vi "17_09_20199_49am.vi"() -> ()   [LabVIEW 2017]
uses:
  <vilib>/Simulation/Scripting/Companion Diagram/SimConfigNode/SimParams.ctl
  <vilib>/Simulation/Scripting/Companion Diagram/SimConfigNode/_simSolvers.ctl
  <vilib>/Simulation/Implementation/Shared/SIMSCR Execution Mode.ctl
  <vilib>/Simulation/Param Hierarchy/Typedefs/SIMPH Param Control Actions.ctl
  <vilib>/Simulation/Implementation/Shared/NILVSim_ParamChanged.vi
  <vilib>/Simulation/Implementation/Shared/NILVSIM_BeginStep.vi
  <vilib>/Simulation/Implementation/Shared/NILVSim_Manager.vi
  <vilib>/Utility/error.llb/Clear Errors.vi
  <vilib>/Simulation/Implementation/Shared/NILVSim_FinalizeModel.vi
  <vilib>/DAQmx/read.llb/DAQmx Read (Counter DBL 1Chan 1Samp).vi
  <vilib>/DAQmx/read.llb/DAQmx Read (Digital Bool 1Line 1Point).vi
  917b7e52-755f-4d44-bea8-9e7c9beac24e.vi
  a58f9967-76f1-4ebc-ad3d-26e75a3ca160.vi
  <vilib>/DAQmx/write.llb/DAQmx Write (Analog DBL 1Chan 1Samp).vi
  <vilib>/DAQmx/create/channels.llb/DAQmx Create Channel (AO-Voltage-Basic).vi
  <vilib>/DAQmx/create/channels.llb/DAQmx Create Channel (DI-Digital Input).vi
  <vilib>/DAQmx/create/channels.llb/DAQmx Create Channel (CI-Count Edges).vi
  <vilib>/Simulation/Implementation/Shared/SIM Unbundle Sim Info.vi
  <vilib>/Simulation/Implementation/Shared/NILVSim_Initialize.vi
  <vilib>/Simulation/Utility/Implementation/NILVSim Get Time and IsAcceptedStep.vi
  <vilib>/Simulation/Implementation/Shared/SIMSH Read Queue.vi
  <vilib>/Simulation/Implementation/Shared/NILVSim_GetModelError.vi
  <vilib>/Simulation/Implementation/Shared/SIM Bundle Sim Info.vi
  Global pulses.vi
  <vilib>/DAQmx/miscellaneous.llb/DAQmx Fill In Error Info.vi
  <vilib>/Simulation/Implementation/XNodeFramework/SimXNode/SimX.xnode
  <vilib>/Simulation/Model Libraries/PID/SIM PID (Parallel).vi
  <vilib>/Simulation/Model Libraries/PID/SIM PID.vi
  <vilib>/Simulation/Scripting/Companion Diagram/SimConfigNode/SimDog.xnode
  <vilib>/Simulation/Model Libraries/PID/SIM PID (Academic).vi
  <vilib>/Simulation/Implementation/Shared/NI_SIM_Implementation.lvlib
panel:
  out "Numeric 2":dbl
  out "swiches pressed y":dbl
  out "swiches pressed x":dbl
  in  "Reset":bool
  out "time":dbl
  out "frequency (moving)":dbl
  out "switch dir":dbl
  out "swiches":bool
  out "Boolean 2":bool
  in  "rectangle":bool
  in  "stage rectangle":T1(ring)
  out "stay1":dbl
  out "stay":dbl
  out "calculating error x":dbl
  out "calculating error y":dbl
  in  "origin":bool
  out "Previous Y":dbl
  out "Previous X":dbl
  out "Current Y":dbl
  out "Current X":dbl
  out "previous index":dbl
  out "both/reset enter":bool
  out "reset complete":bool
  out "x circle":bool
  out "y circle":bool
  out "Point circle is drawing":dbl
  out "false":bool
  in  "Radius 2":dbl
  out "No of Points":dbl
  out "Passing Y":dbl
  out "Y array":dbl[](array[numeric])
  out "array Y length 2":dbl
  out "Passing X":dbl
  out "X array":dbl[](array[numeric])
  out "array x Length 2":dbl
  in  "stage circle":T2(ring)
  in  "check instruc":bool
  out "x entered":dbl
  out "y enetred":dbl
  out "greater -1 x":bool
  out "less 1 x":bool
  out "direction selected":dbl
  out "Shape drawing steps":enum16{"corner", "1st switch", "reverse"}(ring)
  in  "height":dbl
  in  "length":dbl
  in  "Has encoders been reset?":enum16{"don't reset", "reset"}(ring)
  out "x distance currently being travelled":dbl
  out "y distance currently being travelled":dbl
  out "error calced":dbl
  out "p1 dis 2":dbl
  out "p1 dis":dbl
  out "error y":dbl
  out "calc distance y":dbl
  out "calc distanc x":dbl
  out "error x":dbl
  out "reached y":bool
  out "reached x":bool
  out "Numeric":dbl
  out "In drawing mode":bool
  in  "Right-Down":bool
  in  "Left-Up":bool
  in  "Left-Down":bool
  in  "Right-Up":bool
  in  "right":bool
  in  "left":bool
  in  "motor 2":dbl(slide)=1.5 scale=-10.0..10.0
  in  "down":bool
  in  "up":bool
  in  "Y Length":dbl=30.0
  in  "X Length":dbl=30.0
  in  "Motor 2 encoder":tag="Dev1/ctr1"
  out "Pulses M2":dbl format="%.2f"
  in  "Motor 1 encoder":tag="Dev1/ctr0"
  out "Pulses M1":dbl format="%.2f"
  out "Right":bool
  out "Bottom":bool
  out "Left":bool
  out "Top":bool
  in  "Switch 4/Line 3":tag="Dev1/port0/line3"
  in  "Switch 3/Line 2":tag="Dev1/port0/line2"
  in  "Switch 2/Line 1":tag="Dev1/port0/line1"
  in  "Switch 1/Line 0":tag="Dev1/port0/line0"
  in  "Motor stop":bool
  in  "Motor 1":tag="Dev1/ao0"
  in  "max Voltage":dbl=10.0
  in  "Min Voltage":dbl=-10.0
  in  "Motor 2":tag="Dev1/ao1"
  in  "motor 1":dbl(slide)=1.5 scale=-10.0..10.0
  in  "stop":bool
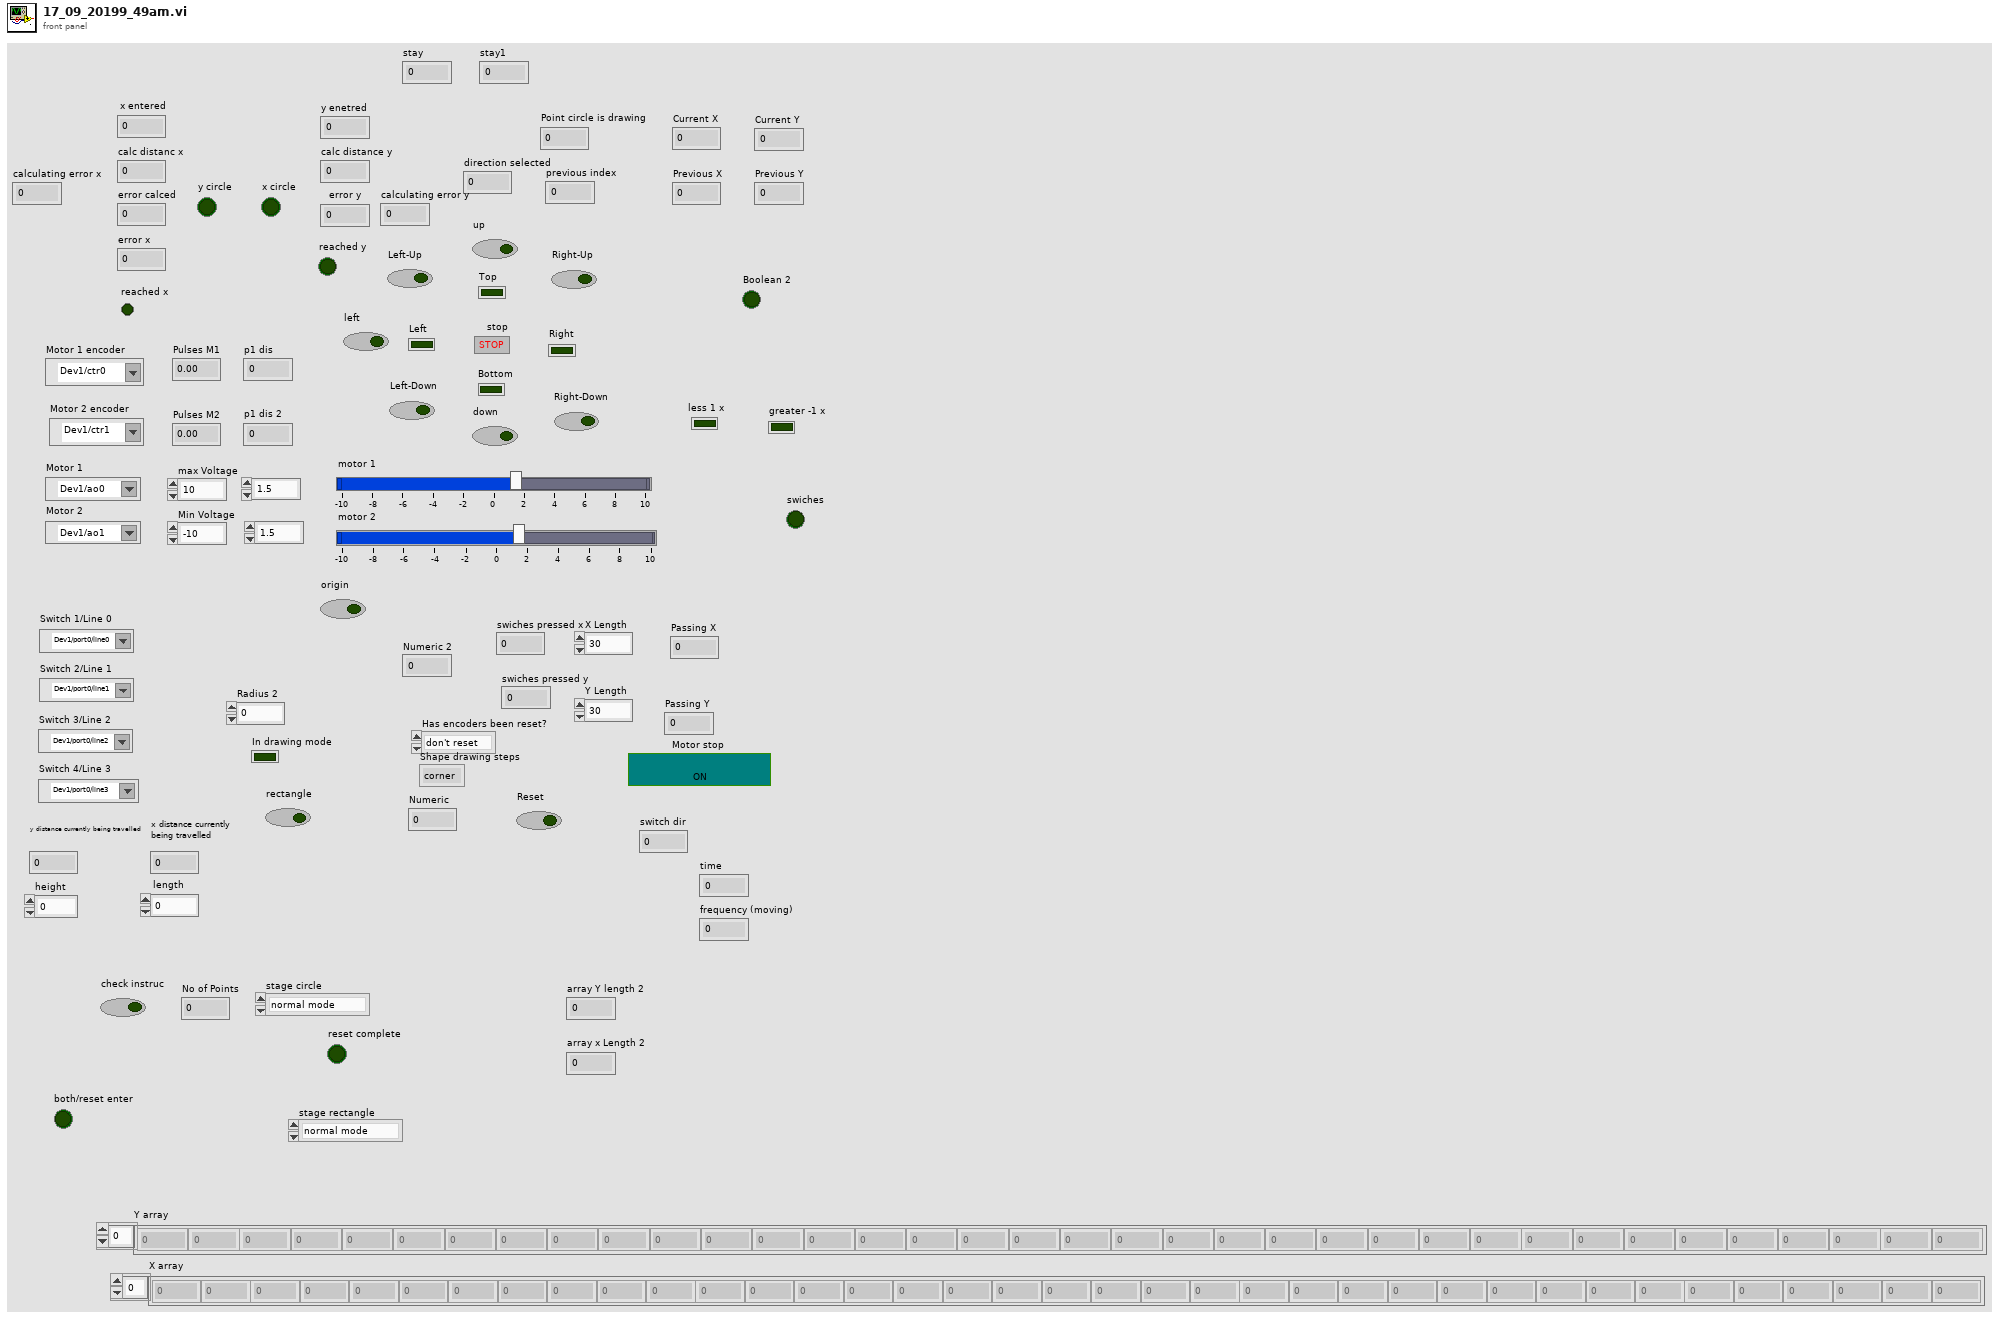
[diagram p1: front panel]
types:
  T1 = enum16{"normal mode", "take to origin", "reset before start", "reset before right", "giving values right", "drawing right", "reset before down", "giving values down", "drawing down", "reset before left", "giving value left", "drawing left", "reset before up", "giving values up", "drawing up", "last step"}
  T2 = enum16{"normal mode", "take to origin", "reset before start", "create points", "draw points", "checking if draw", "reset draw counter"}
  T3 = enum16{"Simulate to Completion", "Single Time-Step Simulation (Fixed Step Only)"}
  T4 = typedef "SIMSCR Execution Mode.ctl" = enum16{"Simulate to Completion", "Single Time-Step Simulation (Fixed Step Only)"}
  T5 = typedef "SIMPH Param Control Actions.ctl" = enum16{"get params", "set params"}
  T6 = cluster{"SIMSH Sim Time":dbl, "SIM PID Derivative Gain.vi":cluster{"output":dbl}, "SIM PID Derivative Gain.vi - SIMSH":cluster{"SIMSH Sim Time":dbl, "t 3":dbl, "Select 2":cluster{"s? t:f":dbl}, "Equal?":cluster{"x = y?":bool}, "Or":cluster{"x .or. y?":bool}, "Equal To 0?":cluster{"x = 0?":bool}}, "High Frequency [s] (Tf)":dbl, "Gain":cluster{"output":dbl}, "Summation":cluster{"Result":dbl}, "Integral Gain - series.vi":cluster{"output":dbl}, "Integral Gain - series.vi - SIMSH":cluster{"SIMSH Sim Time":dbl, "Select 2":cluster{"s? t:f":dbl}, "integral in gain?":bool, "Integrator":cluster{"output y(t)":dbl}, "Gain 2":cluster{"output":dbl}, "Select":cluster{"s? t:f":dbl}, "Equal To 0?":cluster{"x = 0?":bool}, "Reciprocal":cluster{"1/x":dbl}}}
  T7 = typedef "SimParams.ctl" = cluster{"Initial Time (s)":dbl, "Final Time (s)":dbl, "Step Size (s)":dbl, "ODE Solver":T8, "Minimum Step Size (s)":dbl, "Maximum Step Size (s)":dbl, "Relative Tolerance":dbl, "Absolute Tolerance":dbl, "Software Timing":bool, "Initial Step Size (s)":dbl, "Automatic Fixed Step Size?":bool, "Automatic Discrete Step Size?":bool, "Discrete Step Size (s)":dbl, "Calculate using Time Step":bool, "Solver Wired?":bool, "Prev.Frm.Expected End":u64, "Prev.Frm.Actual End":u64, "Prev.Frm.Finished Late?":bool, "Prev.Iter.Expected End":u64, "Prev.Iter.Actual End":u64, "Prev.Iter.Finished Late?":bool, "Expected Iteration Start":u64, "Actual Iteration Start":u64, "Expected Frame Start":u64, "Actual Frame Start":u64, "Source Name":string, "Name":string, "Period":i64, "Deadline":i64, "Offset":i64, "Start":i64, "Priority":i32, "Timeout":i32, "Processor":i32, "Mode":enum32{"No Change", "Process missed periods, maintain original phase", "Discard missed periods, maintain original phase", "Process missed periods, ignore original phase", "Discard missed periods, ignore original phase"}, "Wakeup reason":enum32{"Normal", "Aborted", "Asynchronous wakeup", "Timing source error", "Timed loop error", "Timeout"}, "Error":errorcluster, "Source Type":string, "Secondary Source Type":string, "Global End Time":u64, "Global Start Time":u64, "Full Solver Reset":bool, "Execution Mode":T4, "Nan/Inf Check":bool, "Custom Solver Library":string, "Solver Is Variable":bool, "custom solver name":string, "Signal Collection Decimation":u32}
  T8 = typedef "_simSolvers.ctl" = enum16{"Runge-Kutta 1 (Euler)", "Runge-Kutta 2", "Runge-Kutta 3", "Runge-Kutta 4", "Runge-Kutta 23 (variable)", "Runge-Kutta 45 (variable)", "BDF (variable)", "Adams-Moulton (variable)", "Rosenbrock (variable)", "Discrete States Only", "SDIRK 4 (variable)", "Radau 5 (variable)", "Radau 9 (variable)", "Radau 13 (variable)", "Radau [Variable Order] (variable)", "Gear's Method (variable)", "Linearizer", "State Query", "Trim Eval", "Custom Solver"}
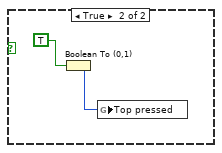
[diagram p2: hidden frame]
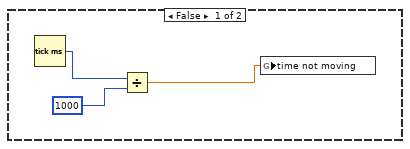
[diagram p6: hidden frame]
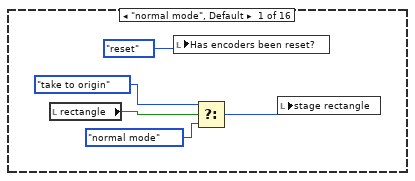
[diagram p8: hidden frame]
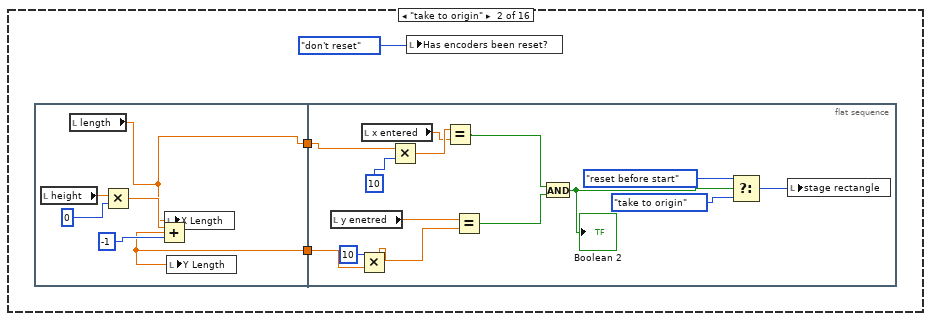
[diagram p9: hidden frame]
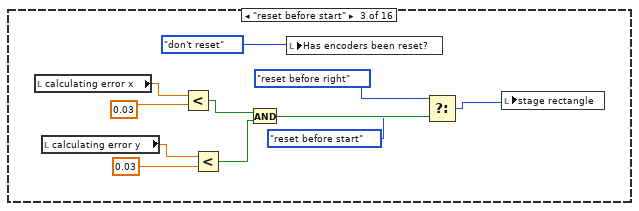
[diagram p10: hidden frame]
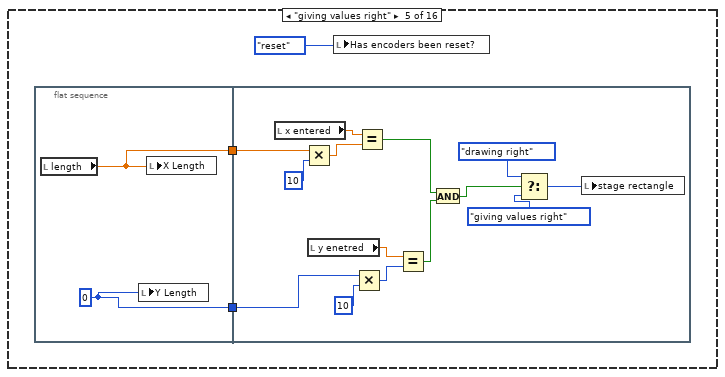
[diagram p11: hidden frame]
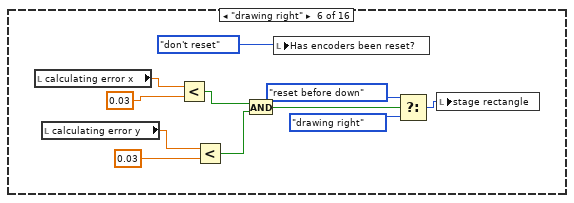
[diagram p12: hidden frame]
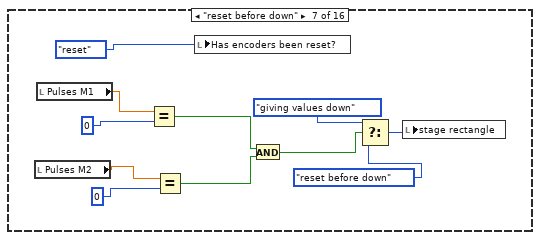
[diagram p13: hidden frame]
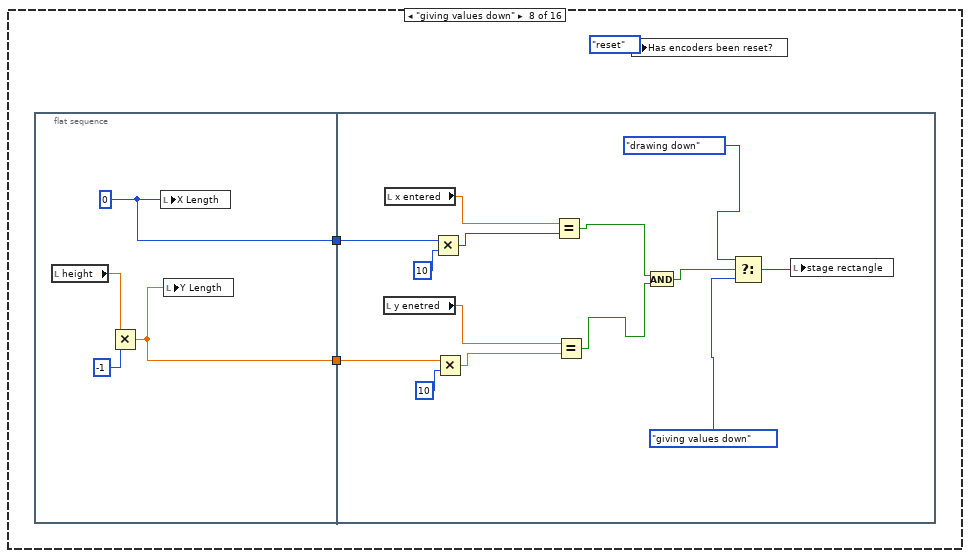
[diagram p14: hidden frame]
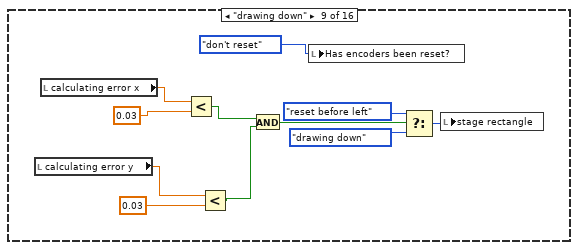
[diagram p15: hidden frame]
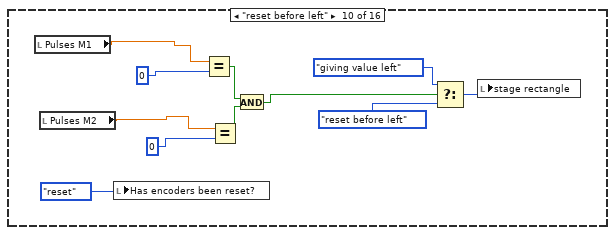
[diagram p16: hidden frame]
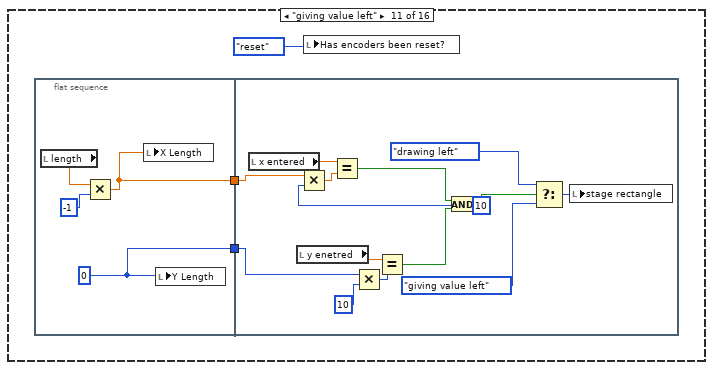
[diagram p17: hidden frame]
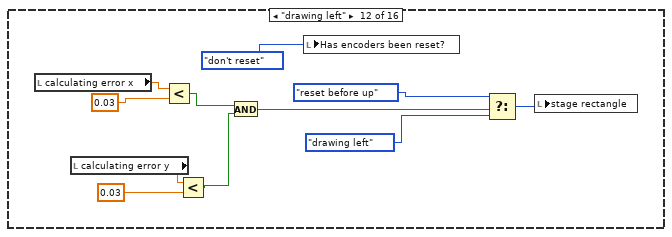
[diagram p18: hidden frame]
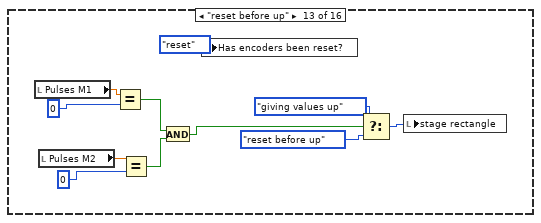
[diagram p19: hidden frame]
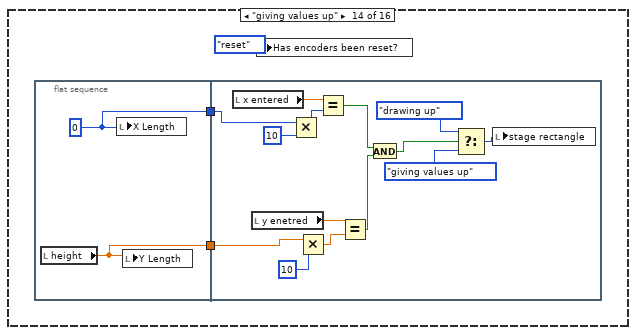
[diagram p20: hidden frame]
diagram:
  n1 = call-poly <vilib>:"DAQmx Create Virtual Channel.vi"("lines"="Switch 1/Line 0") -> ("task out"=w36:refnum<k21>, "error out"=w32:errorcluster)  [unwired: 13 in]
  n2 = call-poly <vilib>:"DAQmx Create Virtual Channel.vi"("lines"="Switch 2/Line 1") -> ("task out"=w35:refnum<k21>, "error out"=w31:errorcluster)  [unwired: 13 in]
  n3 = call-poly <vilib>:"DAQmx Create Virtual Channel.vi"("lines"="Switch 3/Line 2") -> ("task out"=w34:refnum<k21>, "error out"=w30:errorcluster)  [unwired: 13 in]
  n4 = call-poly <vilib>:"DAQmx Create Virtual Channel.vi"("lines"="Switch 4/Line 3") -> ("task out"=w33:refnum<k21>, "error out"=w29:errorcluster)  [unwired: 13 in]
  n5 = call-poly <vilib>:"DAQmx Create Virtual Channel.vi"("maximum value"="max Voltage", "minimum value"="Min Voltage", "physical channels"="Motor 1") -> ("task out"=w46:refnum<k21>, "error out"=w42:errorcluster)  [unwired: 11 in]
  n6 = call <vilib>:"DAQmx Start Task.vi"("task/channels in"=w36, "error in"=w32) -> ("task out"=w28:refnum<k21>, "error out"=w26:errorcluster)  [unwired: 12 in]
  n7 = call <vilib>:"DAQmx Start Task.vi"("task/channels in"=w35, "error in"=w31) -> ("task out"=w24:refnum<k21>, "error out"=w21:errorcluster)  [unwired: 12 in]
  n8 = call-poly <vilib>:"DAQmx Create Virtual Channel.vi"("maximum value"="max Voltage", "minimum value"="Min Voltage", "physical channels"="Motor 2") -> ("task out"=w49:refnum<k21>, "error out"=w41:errorcluster)  [unwired: 11 in]
  n9 = call-poly <vilib>:"DAQmx Create Virtual Channel.vi"("counter"="Motor 1 encoder") -> ("task out"=w7:refnum<k21>, "error out"=w2:errorcluster)  [unwired: 13 in]
  n10 = call-poly <vilib>:"DAQmx Create Virtual Channel.vi"("counter"="Motor 2 encoder") -> ("task out"=w6:refnum<k21>)  [unwired: 13 in, 1 out]
  n11 = call <vilib>:"DAQmx Start Task.vi"("task/channels in"=w34, "error in"=w30) -> ("task out"=w23:refnum<k21>, "error out"=w20:errorcluster)  [unwired: 12 in]
  n12 = call <vilib>:"DAQmx Start Task.vi"("task/channels in"=w33, "error in"=w29) -> ("task out"=w22:refnum<k21>, "error out"=w19:errorcluster)  [unwired: 12 in]
  n13 = call <vilib>:"DAQmx Start Task.vi"("task/channels in"=w7) -> ("task out"=w3:refnum<k21>)  [unwired: 13 in, 1 out]
  n14 = call <vilib>:"DAQmx Start Task.vi"("task/channels in"=w6) -> ("task out"=w1:refnum<k21>)  [unwired: 13 in, 1 out]
  n15 = while {
    tunnel: w49 -> [w249]
    tunnel: [w246] -> w48
    tunnel: w46 -> [w243]
    tunnel: [w242] -> w45
    tunnel: w42 -> [w240]
    tunnel: w41 -> [w239]
    tunnel: w28 -> [w233]
    tunnel: [w232] -> w27
    tunnel: w26 -> [w231]
    tunnel: [w230] -> w25
    tunnel: w24 -> [w229]
    tunnel: w23 -> [w228]
    tunnel: w22 -> [w227]
    tunnel: w21 -> [w226]
    tunnel: w20 -> [w225]
    tunnel: w19 -> [w224]
    tunnel: [w223] -> w18
    tunnel: [w222] -> w17
    tunnel: [w221] -> w16
    tunnel: [w220] -> w15
    tunnel: [w219] -> w14
    tunnel: [w218] -> w13
    tunnel: [w161] -> w10
    tunnel: w3 -> [w163]
    tunnel: w2 -> [w162]
    tunnel: w1 -> [w159]
    stop <- "stop" stop-if-true
    n16 = case shown="True" "check instruc" {
      frame False {
        "false" <- TRUE
      }
      frame True {
        n17 = case shown="\"create points\"" "stage circle" {
          frame "normal mode", Default {
            n18 = local read "check instruc"() -> (w501:bool)
            n19 = local write "Y Length"(0) -> ()
            n20 = local write "X Length"(0) -> ()
            n21 = local write "Has encoders been reset?"(enum16{"don't reset", "reset"}."reset") -> ()
            n22 = Select(t=T2."take to origin", s=w501, f=T2."normal mode") -> (s? t:f=w502:T2)
            n23 = local write "stage circle"(w502) -> ()
          }
          frame "take to origin" {
            n24 = flat-sequence {
              tunnel: [w513] -> w506
              tunnel: [w508] -> w505
              tunnel: w506 -> [w518]
              tunnel: w505 -> [w517]
              frame #0 {
                n25 = local read "Radius 2"() -> (w512:dbl)
                n26 = local read "Radius 2"() -> (w515:dbl)
                n27 = Multiply(x=w512, y=0) -> (x*y=w509:dbl)
                n28 = Multiply(x=w515, y=0) -> (x*y=w513:dbl)
                n29 = Add(x=w509, y=-1) -> (x+y=w508:dbl)
                n30 = local write "Y Length"(w508) -> ()
                n31 = local write "X Length"(w513) -> ()
              }
              frame #1 {
                n32 = Multiply(x=10, y=w517) -> (x*y=w528:dbl)
                n33 = local read "y enetred"() -> (w522:dbl)
                n34 = local read "x entered"() -> (w521:dbl)
                n35 = Multiply(x=10, y=w518) -> (x*y=w527:dbl)
                n36 = Equal?(x=w521, y=w527) -> (x = y?=w524:bool)
                n37 = Equal?(x=w528, y=w522) -> (x = y?=w523:bool)
                n38 = And(x=w524, y=w523) -> (x .and. y?=w529:bool)
                n39 = Select(t=T2."reset before start", s=w529, f=T2."take to origin") -> (s? t:f=w516:T2)
                n40 = local write "stage circle"(w516) -> ()
              }
            }
            n41 = local write "Has encoders been reset?"(enum16{"don't reset", "reset"}."reset") -> ()
          }
          frame "reset before start" {
            n42 = local read "calculating error x"() -> (w539:dbl)
            n43 = local read "calculating error y"() -> (w537:dbl)
            n44 = Less?(x=w539, y=0.01) -> (x < y?=w535:bool)
            n45 = Less?(x=w537, y=0.01) -> (x < y?=w534:bool)
            n46 = local write "Has encoders been reset?"(enum16{"don't reset", "reset"}."don't reset") -> ()
            n47 = And(x=w535, y=w534) -> (x .and. y?=w533:bool)
            n48 = Select(t=T2."create points", s=w533, f=T2."reset before start") -> (s? t:f=w530:T2)
            n49 = local write "stage circle"(w530) -> ()
          }
          frame "create points" {
            n50 = flat-sequence {
              frame #0 {
                n51 = for {
                  N: 36 -> [_]
                  shift-right: [w551] -> w548
                  shift-left: _ -> [_]
                  tunnel: [w551] -> w543 mode=indexing
                  shift-right: [w550] -> w546
                  shift-left: _ -> [_]
                  tunnel: [w550] -> w544 mode=indexing
                  i -> [w552]
                  n52 = Multiply(x=2, y=3.141592653589793) -> (x*y=w555:dbl)
                  n53 = Increment(x=w552) -> (x+1=w553:i32)
                  n54 = Divide(x=w555, y=36) -> (x/y=w557:dbl)
                  n55 = Multiply(x=w557, y=w553) -> (x*y=w554:dbl)
                  n56 = Cosine(x=w554) -> (cos(x)=w560:dbl)
                  n57 = Sine(x=w554) -> (sin(x)=w561:dbl)
                  n58 = Multiply(x=w561, y="Radius 2") -> (x*y=w551:dbl)
                  n59 = Multiply(x=w560, y="Radius 2") -> (x*y=w550:dbl)
                  "No of Points" <- w552
                }
                "Passing Y" <- w548
                "Y array" <- w543
                "Passing X" <- w546
                "X array" <- w544
                n60 = Array Size(array=w543) -> (size(s)=→"array Y length 2":i32)
                n61 = Array Size(array=w544) -> (size(s)=→"array x Length 2":i32)
              }
              frame #1 {
                n62 = local read "Y array"() -> (w568:dbl[])
                n63 = Index Array(array=w568, index=1) -> (element=w569:dbl)
                n64 = local read "X array"() -> (w570:dbl[])
                n65 = Index Array(array=w570, index=1) -> (element=w571:dbl)
                n66 = Insert Into Array(array=w568, index=36, new element=w569) -> (w566:dbl[])
                n67 = Insert Into Array(array=w570, index=36, new element=w571) -> (w567:dbl[])
                n68 = local write "Y array"(w566) -> ()
                n69 = local write "X array"(w567) -> ()
              }
              frame #2 {
                n70 = local read "No of Points"() -> (w576:dbl)
                n71 = Equal?(x=w576, y=35) -> (x = y?=w577:bool)
                n72 = Select(t=T2."draw points", s=w577, f=T2."create points") -> (s? t:f=w575:T2)
                n73 = local write "stage circle"(w575) -> ()
              }
            }
            n74 = local write "Has encoders been reset?"(enum16{"don't reset", "reset"}."don't reset") -> ()
          }
          frame "draw points" {
            n75 = flat-sequence {
              frame #0 {
                n76 = local read "Point circle is drawing"() -> (w606:dbl)
                n77 = local read "previous index"() -> (w598:dbl)
                n78 = local read "Y array"() -> (w599:dbl[])
                n79 = local read "X array"() -> (w600:dbl[])
                n80 = Index Array(array=w599, index=w598) -> (element=→"Previous Y":dbl)
                n81 = Index Array(array=w600, index=w598) -> (element=→"Previous X":dbl)
                n82 = local read "X array"() -> (w601:dbl[])
                n83 = local read "Previous X"() -> (w588:dbl)
                n84 = local read "Current X"() -> (w593:dbl)
                n85 = local read "Y array"() -> (w602:dbl[])
                n86 = local read "Current X"() -> (w591:dbl)
                n87 = Greater Or Equal?(x=w606, y=36) -> (x >= y?=w604:bool)
                n88 = Not Equal To 0?(x=w606) -> (x != 0?=w594:bool)
                n89 = local read "Previous Y"() -> (w589:dbl)
                n90 = local read "Current Y"() -> (w590:dbl)
                n91 = Index Array(array=w601, index=w606) -> (element=→"Current X":dbl)
                n92 = Subtract(x=w591, y=w588) -> (x-y=w586:dbl)
                n93 = Select(t=w586, s=w594, f=w593) -> (s? t:f=w583:dbl)
                n94 = Select(t=T2."normal mode", s=w604, f=T2."draw points") -> (s? t:f=w603:T2)
                n95 = Index Array(array=w602, index=w606) -> (element=→"Current Y":dbl)
                n96 = Subtract(x=w590, y=w589) -> (x-y=w585:dbl)
                n97 = local read "Current Y"() -> (w592:dbl)
                n98 = local write "X Length"(w583) -> ()
                n99 = Not(x=w604) -> (.not. x?=w605:bool)
                n100 = local write "stage circle"(w603) -> ()
                n101 = Not Equal To 0?(x=w606) -> (x != 0?=w595:bool)
                n102 = Select(t=w585, s=w595, f=w592) -> (s? t:f=w584:dbl)
                n103 = local write "Y Length"(w584) -> ()
                n104 = local write "check instruc"(w605) -> ()
              }
              frame #1 {
                n105 = local write "stage circle"(T2."checking if draw") -> ()
              }
            }
            n106 = local write "Has encoders been reset?"(enum16{"don't reset", "reset"}."don't reset") -> ()
          }
          frame "checking if draw" {
            n107 = local read "calculating error x"() -> (w611:dbl)
            n108 = local read "calculating error y"() -> (w609:dbl)
            n109 = local read "Point circle is drawing"() -> (w614:dbl)
            n110 = Greater Or Equal?(x=0.01, y=w611) -> (x >= y?=w617:bool)
            "x circle" <- w617
            n111 = Greater Or Equal?(x=0.01, y=w609) -> (x >= y?=w618:bool)
            "y circle" <- w618
            n112 = And(x=w618, y=w617) -> (x .and. y?=w615:bool)
            "both/reset enter" <- w615
            n113 = Increment(x=w614) -> (x+1=w620:dbl)
            n114 = Select(t=w620, s=w615, f=w614) -> (s? t:f=→"Point circle is drawing":dbl)
            n115 = Select(t=T2."reset draw counter", s=w615, f=T2."checking if draw") -> (s? t:f=w616:T2)
            n116 = local write "stage circle"(w616) -> ()
          }
          frame "reset draw counter" {
            n117 = for {
              N: 1 -> [_]
              i -> [w625]
              n118 = local read "Point circle is drawing"() -> (w630:dbl)
              n119 = local read "Pulses M2"() -> (w635:dbl)
              n120 = local read "Pulses M1"() -> (w636:dbl)
              n121 = Equal To 0?(x=w635) -> (x = 0?=w634:bool)
              n122 = Equal To 0?(x=w636) -> (x = 0?=w632:bool)
              n123 = local read "previous index"() -> (w627:dbl)
              n124 = local write "Has encoders been reset?"(enum16{"don't reset", "reset"}."reset") -> ()
              n125 = And(x=w632, y=w634) -> (x .and. y?=w633:bool)
              n126 = Subtract(x=w630, y=1) -> (x-y=w628:dbl)
              n127 = Select(t=T2."draw points", s=w633, f=T2."reset draw counter") -> (s? t:f=w637:T2)
              n128 = Equal To 0?(x=w625) -> (x = 0?=w624:bool)
              n129 = local write "stage circle"(w637) -> ()
              n130 = Select(t=w628, s=w624, f=w627) -> (s? t:f=→"previous index":dbl)
              "reset complete" <- TRUE
            }
          }
        }
      }
    }
    n131 = case shown="True" "rectangle" {
      frame False {
      }
      frame True {
        n132 = case shown="\"reset before right\"" "stage rectangle" {
          frame "normal mode", Default {
            n133 = local read "rectangle"() -> (w290:bool)
            n134 = local write "Has encoders been reset?"(enum16{"don't reset", "reset"}."reset") -> ()
            n135 = Select(t=T1."take to origin", s=w290, f=T1."normal mode") -> (s? t:f=w288:T1)
            n136 = local write "stage rectangle"(w288) -> ()
          }
          frame "take to origin" {
            n137 = flat-sequence {
              tunnel: [w295] -> w292
              tunnel: [w294] -> w291
              tunnel: w292 -> [w309]
              tunnel: w291 -> [w308]
              frame #0 {
                n138 = local read "height"() -> (w299:dbl)
                n139 = local read "length"() -> (w294:dbl)
                n140 = Multiply(x=w299, y=0) -> (x*y=w297:dbl)
                n141 = Add(x=w297, y=-1) -> (x+y=w295:dbl)
                n142 = local write "X Length"(w294) -> ()
                n143 = local write "Y Length"(w295) -> ()
              }
              frame #1 {
                n144 = local read "y enetred"() -> (w303:dbl)
                n145 = Multiply(x=10, y=w309) -> (x*y=w311:dbl)
                n146 = local read "x entered"() -> (w304:dbl)
                n147 = Multiply(x=w308, y=10) -> (x*y=w307:dbl)
                n148 = Equal?(x=w307, y=w304) -> (x = y?=w306:bool)
                n149 = Equal?(x=w303, y=w311) -> (x = y?=w305:bool)
                n150 = And(x=w306, y=w305) -> (x .and. y?=w313:bool)
                "Boolean 2" <- w313
                n151 = Select(t=T1."reset before start", s=w313, f=T1."take to origin") -> (s? t:f=w302:T1)
                n152 = local write "stage rectangle"(w302) -> ()
              }
            }
            n153 = local write "Has encoders been reset?"(enum16{"don't reset", "reset"}."don't reset") -> ()
          }
          frame "reset before start" {
            n154 = local read "calculating error x"() -> (w318:dbl)
            n155 = local read "calculating error y"() -> (w317:dbl)
            n156 = Less?(x=w318, y=0.03) -> (x < y?=w319:bool)
            n157 = Less?(x=w317, y=0.03) -> (x < y?=w321:bool)
            n158 = And(x=w319, y=w321) -> (x .and. y?=w316:bool)
            n159 = local write "Has encoders been reset?"(enum16{"don't reset", "reset"}."don't reset") -> ()
            n160 = Select(t=T1."reset before right", s=w316, f=T1."reset before start") -> (s? t:f=w323:T1)
            n161 = local write "stage rectangle"(w323) -> ()
          }
          frame "reset before right" {
            n162 = local read "Pulses M2"() -> (w334:dbl)
            n163 = local read "Pulses M1"() -> (w335:dbl)
            n164 = Equal?(x=w335, y=0) -> (x = y?=w333:bool)
            n165 = Equal?(x=w334, y=0) -> (x = y?=w332:bool)
            n166 = And(x=w333, y=w332) -> (x .and. y?=w331:bool)
            n167 = local write "Has encoders been reset?"(enum16{"don't reset", "reset"}."reset") -> ()
            n168 = Select(t=T1."giving values right", s=w331, f=T1."reset before right") -> (s? t:f=w330:T1)
            n169 = local write "stage rectangle"(w330) -> ()
          }
          frame "giving values right" {
            n170 = flat-sequence {
              tunnel: [w339] -> w338
              tunnel: [w340] -> w337
              tunnel: w338 -> [w350]
              tunnel: w337 -> [w349]
              frame #0 {
                w339 = 0
                n171 = local read "length"() -> (w340:dbl)
                n172 = local write "Y Length"(w339) -> ()
                n173 = local write "X Length"(w340) -> ()
              }
              frame #1 {
                n174 = local read "x entered"() -> (w347:dbl)
                n175 = Multiply(x=w349, y=10) -> (x*y=w348:dbl)
                n176 = local read "y enetred"() -> (w345:dbl)
                n177 = Multiply(x=w350, y=10) -> (x*y=w346:i32)
                n178 = Equal?(x=w347, y=w348) -> (x = y?=w352:bool)
                n179 = Equal?(x=w345, y=w346) -> (x = y?=w351:bool)
                n180 = And(x=w352, y=w351) -> (x .and. y?=w343:bool)
                n181 = Select(t=T1."drawing right", s=w343, f=T1."giving values right") -> (s? t:f=w344:T1)
                n182 = local write "stage rectangle"(w344) -> ()
              }
            }
            n183 = local write "Has encoders been reset?"(enum16{"don't reset", "reset"}."reset") -> ()
          }
          frame "drawing right" {
            n184 = local read "calculating error x"() -> (w361:dbl)
            n185 = local read "calculating error y"() -> (w362:dbl)
            n186 = Less?(x=w361, y=0.03) -> (x < y?=w364:bool)
            n187 = Less?(x=w362, y=0.03) -> (x < y?=w365:bool)
            n188 = And(x=w364, y=w365) -> (x .and. y?=w363:bool)
            n189 = local write "Has encoders been reset?"(enum16{"don't reset", "reset"}."don't reset") -> ()
            n190 = Select(t=T1."reset before down", s=w363, f=T1."drawing right") -> (s? t:f=w360:T1)
            n191 = local write "stage rectangle"(w360) -> ()
          }
          frame "reset before down" {
            n192 = local read "Pulses M2"() -> (w370:dbl)
            n193 = local read "Pulses M1"() -> (w371:dbl)
            n194 = Equal?(x=w371, y=0) -> (x = y?=w376:bool)
            n195 = Equal?(x=w370, y=0) -> (x = y?=w375:bool)
            n196 = local write "Has encoders been reset?"(enum16{"don't reset", "reset"}."reset") -> ()
            n197 = And(x=w376, y=w375) -> (x .and. y?=w374:bool)
            n198 = Select(t=T1."giving values down", s=w374, f=T1."reset before down") -> (s? t:f=w367:T1)
            n199 = local write "stage rectangle"(w367) -> ()
          }
          frame "giving values down" {
            n200 = flat-sequence {
              tunnel: [w383] -> w379
              tunnel: [w380] -> w378
              tunnel: w379 -> [w388]
              tunnel: w378 -> [w387]
              frame #0 {
                w383 = 0
                n201 = local read "height"() -> (w382:dbl)
                n202 = Multiply(x=w382, y=-1) -> (x*y=w380:dbl)
                n203 = local write "X Length"(w383) -> ()
                n204 = local write "Y Length"(w380) -> ()
              }
              frame #1 {
                n205 = local read "y enetred"() -> (w389:dbl)
                n206 = local read "x entered"() -> (w390:dbl)
                n207 = Multiply(x=w388, y=10) -> (x*y=w396:i32)
                n208 = Multiply(x=w387, y=10) -> (x*y=w394:dbl)
                n209 = Equal?(x=w390, y=w396) -> (x = y?=w391:bool)
                n210 = Equal?(x=w389, y=w394) -> (x = y?=w392:bool)
                n211 = And(x=w391, y=w392) -> (x .and. y?=w393:bool)
                n212 = Select(t=T1."drawing down", s=w393, f=T1."giving values down") -> (s? t:f=w384:T1)
                n213 = local write "stage rectangle"(w384) -> ()
              }
            }
            n214 = local write "Has encoders been reset?"(enum16{"don't reset", "reset"}."reset") -> ()
          }
          frame "drawing down" {
            n215 = local read "calculating error y"() -> (w403:dbl)
            n216 = local read "calculating error x"() -> (w402:dbl)
            n217 = Less?(x=w402, y=0.03) -> (x < y?=w407:bool)
            n218 = Less?(x=w403, y=0.03) -> (x < y?=w408:bool)
            n219 = And(x=w407, y=w408) -> (x .and. y?=w406:bool)
            n220 = local write "Has encoders been reset?"(enum16{"don't reset", "reset"}."don't reset") -> ()
            n221 = Select(t=T1."reset before left", s=w406, f=T1."drawing down") -> (s? t:f=w399:T1)
            n222 = local write "stage rectangle"(w399) -> ()
          }
          frame "reset before left" {
            n223 = local read "Pulses M1"() -> (w415:dbl)
            n224 = local read "Pulses M2"() -> (w414:dbl)
            n225 = local write "Has encoders been reset?"(enum16{"don't reset", "reset"}."reset") -> ()
            n226 = Equal?(x=w415, y=0) -> (x = y?=w419:bool)
            n227 = Equal?(x=w414, y=0) -> (x = y?=w418:bool)
            n228 = And(x=w419, y=w418) -> (x .and. y?=w413:bool)
            n229 = Select(t=T1."giving value left", s=w413, f=T1."reset before left") -> (s? t:f=w410:T1)
            n230 = local write "stage rectangle"(w410) -> ()
          }
          frame "giving value left" {
            n231 = flat-sequence {
              tunnel: [w426] -> w422
              tunnel: [w423] -> w421
              tunnel: w422 -> [w436]
              tunnel: w421 -> [w435]
              frame #0 {
                w426 = 0
                n232 = local read "length"() -> (w424:dbl)
                n233 = Multiply(x=w424, y=-1) -> (x*y=w423:dbl)
                n234 = local write "X Length"(w423) -> ()
                n235 = local write "Y Length"(w426) -> ()
              }
              frame #1 {
                n236 = local read "x entered"() -> (w434:dbl)
                n237 = local read "y enetred"() -> (w433:dbl)
                n238 = Multiply(x=w435, y=10) -> (x*y=w439:dbl)
                n239 = Equal?(x=w434, y=w439) -> (x = y?=w431:bool)
                n240 = Multiply(x=w436, y=10) -> (x*y=w437:i32)
                n241 = Equal?(x=w433, y=w437) -> (x = y?=w430:bool)
                n242 = And(x=w431, y=w430) -> (x .and. y?=w432:bool)
                n243 = Select(t=T1."drawing left", s=w432, f=T1."giving value left") -> (s? t:f=w427:T1)
                n244 = local write "stage rectangle"(w427) -> ()
              }
            }
            n245 = local write "Has encoders been reset?"(enum16{"don't reset", "reset"}."reset") -> ()
          }
          frame "drawing left" {
            n246 = local read "calculating error x"() -> (w445:dbl)
            n247 = local read "calculating error y"() -> (w446:dbl)
            n248 = Less?(x=w445, y=0.03) -> (x < y?=w450:bool)
            n249 = Less?(x=w446, y=0.03) -> (x < y?=w451:bool)
            n250 = And(x=w450, y=w451) -> (x .and. y?=w449:bool)
            n251 = local write "Has encoders been reset?"(enum16{"don't reset", "reset"}."don't reset") -> ()
            n252 = Select(t=T1."reset before up", s=w449, f=T1."drawing left") -> (s? t:f=w442:T1)
            n253 = local write "stage rectangle"(w442) -> ()
          }
          frame "reset before up" {
            n254 = local read "Pulses M1"() -> (w457:dbl)
            n255 = local read "Pulses M2"() -> (w456:dbl)
            n256 = Equal?(x=w457, y=0) -> (x = y?=w462:bool)
            n257 = Equal?(x=w456, y=0) -> (x = y?=w461:bool)
            n258 = And(x=w462, y=w461) -> (x .and. y?=w458:bool)
            n259 = local write "Has encoders been reset?"(enum16{"don't reset", "reset"}."reset") -> ()
            n260 = Select(t=T1."giving values up", s=w458, f=T1."reset before up") -> (s? t:f=w453:T1)
            n261 = local write "stage rectangle"(w453) -> ()
          }
          frame "giving values up" {
            n262 = flat-sequence {
              tunnel: [w467] -> w465
              tunnel: [w466] -> w464
              tunnel: w465 -> [w477]
              tunnel: w464 -> [w476]
              frame #0 {
                w466 = 0
                n263 = local read "height"() -> (w467:dbl)
                n264 = local write "X Length"(w466) -> ()
                n265 = local write "Y Length"(w467) -> ()
              }
              frame #1 {
                n266 = local read "x entered"() -> (w479:dbl)
                n267 = local read "y enetred"() -> (w478:dbl)
                n268 = Multiply(x=w476, y=10) -> (x*y=w481:i32)
                n269 = Multiply(x=w477, y=10) -> (x*y=w480:dbl)
                n270 = Equal?(x=w479, y=w481) -> (x = y?=w474:bool)
                n271 = Equal?(x=w478, y=w480) -> (x = y?=w473:bool)
                n272 = And(x=w474, y=w473) -> (x .and. y?=w475:bool)
                n273 = Select(t=T1."drawing up", s=w475, f=T1."giving values up") -> (s? t:f=w470:T1)
                n274 = local write "stage rectangle"(w470) -> ()
              }
            }
            n275 = local write "Has encoders been reset?"(enum16{"don't reset", "reset"}."reset") -> ()
          }
          frame "drawing up" {
            n276 = local read "calculating error x"() -> (w487:dbl)
            n277 = local read "calculating error y"() -> (w486:dbl)
            n278 = Less?(x=w487, y=0.03) -> (x < y?=w491:bool)
            n279 = Less?(x=w486, y=0.03) -> (x < y?=w492:bool)
            n280 = And(x=w491, y=w492) -> (x .and. y?=w490:bool)
            n281 = Select(t=T1."last step", s=w490, f=T1."drawing up") -> (s? t:f=w483:T1)
            n282 = local write "Has encoders been reset?"(enum16{"don't reset", "reset"}."don't reset") -> ()
            n283 = local write "stage rectangle"(w483) -> ()
          }
          frame "last step" {
            n284 = local write "X Length"(0) -> ()
            n285 = local write "Y Length"(0) -> ()
            n286 = local write "Has encoders been reset?"(enum16{"don't reset", "reset"}."reset") -> ()
          }
        }
      }
    }
    n287 = local read "y enetred"() -> (w93:dbl)
    n288 = local read "calc distance y"() -> (w92:dbl)
    n289 = local read "calc distanc x"() -> (w91:dbl)
    n290 = local read "x entered"() -> (w90:dbl)
    n291 = local read "stay"() -> (w87:dbl)
    n292 = local read "stay1"() -> (w86:dbl)
    n293 = formula code="if (Ylength==0)\nYerror=0;\n else  \nif(Ylength<0)\nYerror= Ylength+calculating_y_dis;\nelse\nYerror= Ylength-calculating_y_dis;\n\nif (stay==0)\nYerror=0;"("Ylength"=w93, "calculating_y_dis"=w92, "stay"=w87) -> ("Yerror"=→"error y":dbl)
    n294 = formula code="if (desired_xlength==0)\nXerror=0;\nelse\nif(desired_xlength>0)\nXerror=desired_xlength-actual_xLength;\nelse\nXerror=desired_xlength+actual_xLength;\n\nif (stay1==0)\nXerror=0;"("desired_xlength"=w90, "actual_xLength"=w91, "stay1"=w86) -> ("Xerror"=→"error x":dbl)
    n295 = local read "error y"() -> (w134:dbl)
    n296 = local read "error y"() -> (w133:dbl)
    n297 = local read "error x"() -> (w135:dbl)
    n298 = local read "error y"() -> (w148:dbl)
    n299 = local read "error y"() -> (w146:dbl)
    n300 = local read "error x"() -> (w142:dbl)
    n301 = local read "error x"() -> (w141:dbl)
    n302 = local read "error y"() -> (w149:dbl)
    n303 = local read "error x"() -> (w150:dbl)
    n304 = Less Than 0?(x=w134) -> (x < 0?=w132:bool)
    n305 = Less Than 0?(x=w135) -> (x < 0?=w131:bool)
    n306 = Greater Than 0?(x=w133) -> (x > 0?=w130:bool)
    n307 = Less Than 0?(x=w146) -> (x < 0?=w144:bool)
    n308 = Equal To 0?(x=w150) -> (x = 0?=w145:bool)
    n309 = Greater Than 0?(x=w148) -> (x > 0?=w147:bool)
    n310 = local read "error y"() -> (w127:dbl)
    n311 = local read "error x"() -> (w126:dbl)
    n312 = Greater Than 0?(x=w142) -> (x > 0?=w140:bool)
    n313 = Equal To 0?(x=w149) -> (x = 0?=w139:bool)
    n314 = Less Than 0?(x=w141) -> (x < 0?=w138:bool)
    n315 = And(x=w132, y=w131) -> (x .and. y?=w128:bool)
    n316 = And(x=w131, y=w130) -> (x .and. y?=w129:bool)
    n317 = And(x=w147, y=w145) -> (x .and. y?=w69:bool)
    n318 = And(x=w145, y=w144) -> (x .and. y?=w143:bool)
    n319 = local read "error y"() -> (w122:dbl)
    n320 = And(x=w140, y=w139) -> (x .and. y?=w137:bool)
    n321 = And(x=w139, y=w138) -> (x .and. y?=w136:bool)
    n322 = Greater Than 0?(x=w127) -> (x > 0?=w125:bool)
    n323 = Greater Than 0?(x=w126) -> (x > 0?=w123:bool)
    n324 = Less Than 0?(x=w122) -> (x < 0?=w121:bool)
    n325 = And(x=w125, y=w123) -> (x .and. y?=w124:bool)
    n326 = And(x=w123, y=w121) -> (x .and. y?=w120:bool)
    n327 = Select(t=1, s=w69, f=0) -> (s? t:f=w204:i32)
    n328 = Select(t=10, s=w136, f=0) -> (s? t:f=w202:i32)
    n329 = Select(t=2, s=w143, f=0) -> (s? t:f=w203:i32)
    n330 = Select(t=100, s=w124, f=0) -> (s? t:f=w200:i32)
    n331 = Select(t=200, s=w128, f=0) -> (s? t:f=w199:i32)
    n332 = Select(t=20, s=w137, f=0) -> (s? t:f=w201:i32)
    n333 = Select(t=1000, s=w129, f=0) -> (s? t:f=w198:i32)
    n334 = Select(t=2000, s=w120, f=0) -> (s? t:f=w184:i32)
    n335 = Add(x=w204, y=w203) -> (x+y=w197:i32)
    n336 = Add(x=w202, y=w201) -> (x+y=w196:i32)
    n337 = Add(x=w200, y=w199) -> (x+y=w195:i32)
    n338 = Add(x=w198, y=w184) -> (x+y=w183:i32)
    n339 = Add(x=w197, y=w196) -> (x+y=w194:i32)
    n340 = Add(x=w195, y=w183) -> (x+y=w182:i32)
    n341 = call-poly <vilib>:"DAQmx Read.vi"("task/channels in"=w233, "error in"=w231) -> ("task out"=w232:refnum<k21>, "data"=w53:bool, "error out"=w230:errorcluster)  [unwired: 11 in]
    "Top" <- w53
    n342 = call-poly <vilib>:"DAQmx Read.vi"("task/channels in"=w229, "error in"=w226) -> ("task out"=w223:refnum<k21>, "data"=w68:bool, "error out"=w220:errorcluster)  [unwired: 11 in]
    "Bottom" <- w68
    n343 = call-poly <vilib>:"DAQmx Read.vi"("task/channels in"=w228, "error in"=w225) -> ("task out"=w222:refnum<k21>, "data"=w67:bool, "error out"=w219:errorcluster)  [unwired: 11 in]
    "Right" <- w67
    n344 = local read "Pulses M2"() -> (w164:dbl)
    n345 = call-poly <vilib>:"DAQmx Read.vi"("task/channels in"=w227, "error in"=w224) -> ("task out"=w221:refnum<k21>, "data"=w66:bool, "error out"=w218:errorcluster)  [unwired: 11 in]
    "Left" <- w66
    n346 = local read "Numeric 2"() -> (w55:dbl)
    n347 = local read "Pulses M1"() -> (w160:dbl)
    n348 = Add(x=w194, y=w182) -> (x+y=w58:i32)
    "direction selected" <- w58
    n349 = case shown="1" w55 {
      selector: w55 -> [_ w257]
      frame 0, Default {
      }
      frame 1 {
        n350 = local read "calculating error y"() -> (w258:dbl)
        n351 = local read "swiches pressed x"() -> (w253:dbl)
        n352 = local read "swiches pressed y"() -> (w254:dbl)
        n353 = formula code="if (swiches=1)\nstay=1;\nXlength=x;\nYlength=y;\nif(Yerror==0)\nstay=0;"("stay"=1.0 ("input variable"), "Yerror"=w258, "swiches"=w257, "x"=w253, "y"=w254) -> ("Xlength"=w256:dbl, "Ylength"=w255:dbl)
        n354 = local write "X Length"(w256) -> ()
        n355 = local write "Y Length"(w255) -> ()
      }
    }
    n356 = local read "reached y"() -> (w60:bool)
    n357 = local read "reached x"() -> (w61:bool)
    n358 = Multiply(x="Y Length", y=10) -> (x*y=w107:dbl)
    "y enetred" <- w107
    n359 = Divide(x=w160, y=52.56) -> (x/y=→"p1 dis":dbl)
    n360 = Not And(1:w60, 2:w61) -> (0:w59:bool)
    n361 = feedback #1() -> (w104:dbl)  [unwired: 1 in]
    "calc distance y" <- w104
    n362 = formula code="Yerror=  (abs(Ylength)- abs(calculating_y_dis));\nif (Yerror<0.01)\nstay=0;\nif (stay==0)\nYerror=0;"("Ylength"=w107, "calculating_y_dis"=w104, "stay"=1) -> ("Yerror"=w152:dbl, "stay"=→"stay":i32)
    n363 = case shown="True" "Reset" {
      frame False {
      }
      frame True {
        n364 = local write "Has encoders been reset?"(enum16{"don't reset", "reset"}."reset") -> ()
        n365 = local write "Numeric 2"(0) -> ()
      }
    }
    n366 = Divide(x=w164, y=52.56) -> (x/y=→"p1 dis 2":dbl)
    n367 = formula code="X=((PulseM1/52.56)+(PulseM2/52.56))/2.0;\nY=((PulseM1/52.56)+(PulseM2/52.56))/2.0;"("PulseM1"=w160, "PulseM2"=w164) -> ("X"=w77:dbl, "Y"=w78:dbl)
    "calc distanc x" <- w77
    n368 = feedback-in #1(w78) -> ()
    n369 = case shown="True" w59 {
      frame False {
        n370 = Tick Count (ms)() -> (millisecond timer value=w264:u32)
        n371 = Divide(x=w264, y=1000) -> (x/y=w262:dbl)
        n372 = global write "Global pulses.vi" "time not moving"(w262) -> ()
      }
      frame True {
        n373 = global read "Global pulses.vi" "Time variable"() -> (→"time":dbl)
        n374 = local read "Pulses M1"() -> (w282:dbl)
        n375 = local read "Pulses M2"() -> (w283:dbl)
        n376 = global read "Global pulses.vi" "Frequency"() -> (→"frequency (moving)":dbl)
        n377 = Tick Count (ms)() -> (millisecond timer value=w275:u32)
        n378 = global read "Global pulses.vi" "Time variable"() -> (w280:dbl)
        n379 = global read "Global pulses.vi" "Enc M2"() -> (w281:dbl)
        n380 = global read "Global pulses.vi" "Time variable"() -> (w279:dbl)
        n381 = global write "Global pulses.vi" "Enc M2"(w283) -> ()
        n382 = global read "Global pulses.vi" "Enc M1"() -> (w278:dbl)
        n383 = Divide(x=w275, y=1000) -> (x/y=w265:dbl)
        n384 = global read "Global pulses.vi" "time not moving"() -> (w266:dbl)
        n385 = Divide(x=w278, y=w279) -> (x/y=w276:dbl)
        n386 = Divide(x=w281, y=w280) -> (x/y=w277:dbl)
        n387 = global write "Global pulses.vi" "Enc M1"(w282) -> ()
        n388 = global read "Global pulses.vi" "Frequncy M1"() -> (w272:dbl)
        n389 = global write "Global pulses.vi" "Frequncy M1"(w276) -> ()
        n390 = global read "Global pulses.vi" "Frequency M2"() -> (w271:dbl)
        n391 = global write "Global pulses.vi" "Frequency M2"(w277) -> ()
        n392 = Subtract(x=w265, y=w266) -> (x-y=w267:dbl)
        n393 = Add(x=w272, y=w271) -> (x+y=w269:dbl)
        n394 = global write "Global pulses.vi" "Time variable"(w267) -> ()
        n395 = Divide(x=w269, y=2) -> (x/y=w268:dbl)
        n396 = global write "Global pulses.vi" "Frequency"(w268) -> ()
      }
    }
    n397 = xnode "PID"("Error"=w152) -> ("Output"=w100:dbl)  [unwired: 2 in, 11 out]
    n398 = Multiply(x="X Length", y=10) -> (x*y=w110:dbl)
    "x entered" <- w110
    n399 = Greater?(x=w100, y=-0.01) -> (0:w97:bool)
    n400 = Less?(x=w100, y=0.01) -> (x < y?=w96:bool)
    n401 = case shown="False" w53 {
      frame False {
      }
      frame True {
        n402 = Boolean To (0,1)(Boolean=TRUE) -> (0, 1=w250:i16)
        n403 = global write "Global pulses.vi" "Top pressed"(w250) -> ()
      }
    }
    n404 = case shown="2" w58 {
      tunnel: "motor 1" -> [w1190 w1193 w1196 w1203 w1207 w1211 w1217 w1223 w1229 w1234 w1241]
      tunnel: "motor 2" -> [w1187 w1195 w1198 w1201 w1206 w1209 w1215 w1221 w1227 w1235 w1240]
      tunnel: [w1186 w1195 w1197 w1200 w1206 w1208 w1214 w1220 w1226 w1232 w1239] -> w108
      tunnel: [w1189 w1192 w1196 w1202 w1207 w1210 w1216 w1222 w1228 w1233 w1238] -> w109
      frame 0, Default {
        n405 = Multiply(x=0, y=w1190) -> (x*y=w1189:dbl)
        n406 = Multiply(x=0, y=w1187) -> (x*y=w1186:dbl)
      }
      frame 1 {
        n407 = Multiply(x=-1, y=w1193) -> (x*y=w1192:dbl)
      }
      frame 2 {
        n408 = Multiply(x=-1.03, y=w1198) -> (x*y=w1197:dbl)
      }
      frame 10 {
        n409 = Multiply(x=-1, y=w1203) -> (x*y=w1202:dbl)
        n410 = Multiply(x=-1.1, y=w1201) -> (x*y=w1200:dbl)
      }
      frame 20 {
      }
      frame 100 {
        n411 = Multiply(x=0, y=w1211) -> (x*y=w1210:dbl)
        n412 = Multiply(x=1, y=w1209) -> (x*y=w1208:dbl)
      }
      frame 200 {
        n413 = Multiply(x=0, y=w1217) -> (x*y=w1216:dbl)
        n414 = Multiply(x=-1, y=w1215) -> (x*y=w1214:dbl)
      }
      frame 1000 {
        n415 = Multiply(x=-1, y=w1223) -> (x*y=w1222:dbl)
        n416 = Multiply(x=0, y=w1221) -> (x*y=w1220:dbl)
      }
      frame 2000 {
        n417 = Multiply(x=1, y=w1229) -> (x*y=w1228:dbl)
        n418 = Multiply(x=0, y=w1227) -> (x*y=w1226:dbl)
      }
      frame 4000 {
        n419 = Multiply(x=-1, y=w1234) -> (x*y=w1233:dbl)
        n420 = Multiply(x=0, y=w1235) -> (x*y=w1232:dbl)
      }
      frame 8000 {
        n421 = Multiply(x=-1, y=w1241) -> (x*y=w1238:dbl)
        n422 = Multiply(x=0, y=w1240) -> (x*y=w1239:dbl)
      }
    }
    n423 = formula code="Xerror=(abs(desired_xlength)-abs(actual_xLength));\n\nif (Xerror<0.01)\nstay1 =0;\nif (stay1==0)\nXerror=0;"("actual_xLength"=w77, "desired_xlength"=w110, "stay1"=1) -> ("Xerror"=w151:dbl, "stay1"=→"stay1":i32)
    "error calced" <- w151
    n424 = local read "Numeric"() -> (w154:dbl)
    n425 = And(x=w97, y=w96) -> (x .and. y?=w115:bool)
    "reached y" <- w115
    n426 = Multiply(x=0, y=w100) -> (x*y=w119:dbl)
    n427 = Or(x=w53, y=w68) -> (x .or. y?=w65:bool)
    n428 = Or(x=w67, y=w66) -> (x .or. y?=w64:bool)
    n429 = Select(t=w119, s=w115, f=w100) -> (s? t:f=→"calculating error y":dbl)
    n430 = And(x=w66, y=w53) -> (x .and. y?=w155:bool)
    n431 = local read "Reset"() -> (w158:bool)
    n432 = local read "rectangle"() -> (w157:bool)
    n433 = Or(x=w65, y=w64) -> (x .or. y?=w54:bool)
    "swiches" <- w54
    n434 = case shown="True" w54 {
      frame False {
      }
      frame True {
        "Numeric 2" <- 1
      }
    }
    n435 = Exclusive Or(1:w53, 2:w66) -> (0:w180:bool)
    n436 = Select(t=1, s=w66, f=0) -> (s? t:f=w169:i32)
    n437 = Select(t=2, s=w53, f=w169) -> (s? t:f=w173:i32)
    n438 = local read "check instruc"() -> (w103:bool)
    n439 = local read "Has encoders been reset?"() -> (w105:enum16{"don't reset", "reset"})
    n440 = xnode "PID 2"("Error"=w151) -> ("Output"=w99:dbl)  [unwired: 2 in, 11 out]
    n441 = Or(x=w158, y=w157) -> (x .or. y?=w102:bool)
    n442 = Select(t=1, s=w180, f=w154) -> (s? t:f=w179:dbl)
    n443 = Select(t=2, s=w155, f=w179) -> (s? t:f=w177:dbl)
    n444 = Greater?(x=w99, y=-0.01) -> (0:w113:bool)
    "greater -1 x" <- w113
    n445 = local read "origin"() -> (w70:bool)
    n446 = Or(x=w102, y=w103) -> (x .or. y?=w101:bool)
    n447 = call "Number To Enum.vim"("number"=w173, "enum type"=enum16{"Nothing", "Left", "Top"}."Nothing") -> ("number as enum"=w170:enum16{"Nothing", "Left", "Top"})
    n448 = case shown="True" "origin" {
      selector: "origin" -> [w1163 w1171]
      tunnel: [w1163 w1171] -> w181
      tunnel: w170 -> [_ w1164]
      frame False {
      }
      frame True {
        n449 = local read "Numeric"() -> (w1169:dbl)
        n450 = local read "Shape drawing steps"() -> (w1166:enum16{"corner", "1st switch", "reverse"})
        n451 = Equal?(x=w1169, y=2) -> (x = y?=w1168:bool)
        n452 = Select(t=enum16{"corner", "1st switch", "reverse"}."reverse", s=w1168, f=w1166) -> (s? t:f=w1165:enum16{"corner", "1st switch", "reverse"})
        n453 = case shown="\"1st switch\"" w1165 {
          tunnel: w1164 -> [_ w1175 _]
          frame "corner" {
            n454 = local write "Y Length"(50) -> ()
            n455 = local write "Has encoders been reset?"(enum16{"don't reset", "reset"}."don't reset") -> ()
            n456 = local write "X Length"(-50) -> ()
          }
          frame "1st switch" {
            n457 = case shown="\"Left\"" w1175 {
              frame "Nothing", Default {
                n458 = local write "Y Length"(0) -> ()
                n459 = local write "X Length"(0) -> ()
                n460 = local write "Numeric"(2) -> ()
              }
              frame "Left" {
                n461 = local write "X Length"(0) -> ()
                n462 = local write "Y Length"(50) -> ()
              }
              frame "Top" {
                n463 = local write "X Length"(-50) -> ()
                n464 = local write "Y Length"(0) -> ()
              }
            }
            n465 = local write "Has encoders been reset?"(enum16{"don't reset", "reset"}."don't reset") -> ()
          }
          frame "reverse" {
            n466 = local write "Has encoders been reset?"(enum16{"don't reset", "reset"}."reset") -> ()
            "Numeric" <- 2
          }
        }
      }
    }
    "In drawing mode" <- w181
    n467 = Less?(x=w99, y=0.01) -> (x < y?=w114:bool)
    "less 1 x" <- w114
    n468 = case shown="True" w101 {
      tunnel: w163 -> [w651 w656]
      tunnel: w162 -> [w652 w655]
      tunnel: [w649 w654] -> w161
      frame False {
        n469 = call-poly <vilib>:"DAQmx Read.vi"("task/channels in"=w651, "error in"=w652) -> ("data"=w650:dbl, "error out"=w649:errorcluster)  [unwired: 11 in, 1 out]
        n470 = local write "Pulses M1"(w650) -> ()
      }
      frame True {
        n471 = case shown="\"don't reset\", Default" "Has encoders been reset?" {
          tunnel: w656 -> [w660 w667]
          tunnel: w655 -> [w659 w666]
          tunnel: [w657 w668] -> w654
          frame "don't reset", Default {
            n472 = call-poly <vilib>:"DAQmx Read.vi"("task/channels in"=w660, "error in"=w659) -> ("data"=→"Pulses M1":dbl, "error out"=w657:errorcluster)  [unwired: 11 in, 1 out]
          }
          frame "reset" {
            n473 = call <vilib>:"DAQmx Stop Task.vi"("task/channels in"=w667, "error in"=w666) -> ("task out"=w665:refnum<k21>, "error out"=w664:errorcluster)  [unwired: 12 in]
            n474 = call <vilib>:"DAQmx Start Task.vi"("task/channels in"=w665, "error in"=w664) -> ("task out"=w663:refnum<k21>, "error out"=w662:errorcluster)  [unwired: 12 in]
            n475 = call-poly <vilib>:"DAQmx Read.vi"("task/channels in"=w663, "error in"=w662) -> ("data"=w661:dbl, "error out"=w668:errorcluster)  [unwired: 11 in, 1 out]
            n476 = local write "Pulses M1"(w661) -> ()
          }
        }
      }
    }
    n477 = case shown="True" w101 {
      tunnel: w159 -> [w640 w642]
      tunnel: w105 -> [_ w641]
      frame False {
        n478 = call-poly <vilib>:"DAQmx Read.vi"("task/channels in"=w640) -> ("data"=w639:dbl)  [unwired: 12 in, 2 out]
        n479 = local write "Pulses M2"(w639) -> ()
      }
      frame True {
        n480 = case shown="\"reset\"" w641 {
          tunnel: w642 -> [w644 w647]
          frame "don't reset", Default {
            n481 = call-poly <vilib>:"DAQmx Read.vi"("task/channels in"=w644) -> ("data"=→"Pulses M2":dbl)  [unwired: 12 in, 2 out]
          }
          frame "reset" {
            n482 = call <vilib>:"DAQmx Stop Task.vi"("task/channels in"=w647) -> ("task out"=w646:refnum<k21>)  [unwired: 13 in, 1 out]
            n483 = call <vilib>:"DAQmx Start Task.vi"("task/channels in"=w646) -> ("task out"=w648:refnum<k21>)  [unwired: 13 in, 1 out]
            n484 = call-poly <vilib>:"DAQmx Read.vi"("task/channels in"=w648) -> ("data"=w645:dbl)  [unwired: 12 in, 2 out]
            n485 = local write "Pulses M2"(w645) -> ()
          }
        }
      }
    }
    n486 = call "Number To Enum.vim"("number"=w177, "enum type"=enum16{"corner", "1st switch", "reverse"}."corner") -> ("number as enum"=→"Shape drawing steps":enum16{"corner", "1st switch", "reverse"})
    n487 = Boolean To (0,1)(Boolean=w66) -> (0, 1=w72:i16)
    n488 = Boolean To (0,1)(Boolean=w70) -> (0, 1=w71:i16)
    n489 = Boolean To (0,1)(Boolean=w53) -> (0, 1=w75:i16)
    n490 = Boolean To (0,1)(Boolean=w67) -> (0, 1=w73:i16)
    n491 = Boolean To (0,1)(Boolean=w68) -> (0, 1=w74:i16)
    n492 = Multiply(x=0, y=w99) -> (x*y=w117:dbl)
    n493 = And(x=w113, y=w114) -> (x .and. y?=w63:bool)
    "reached x" <- w63
    n494 = And(x=w115, y=w63) -> (x .and. y?=w76:bool)
    n495 = Or(x=w76, y="Motor stop") -> (x .or. y?=w217:bool)
    n496 = Or(x=w217, y="stop") -> (x .or. y?=w237:bool)
    n497 = Select(t=0.0, s=w237, f=w108) -> (s? t:f=w234:dbl)
    n498 = call-poly <vilib>:"DAQmx Write.vi"("task/channels in"=w243, "data"=w234, "error in"=w240) -> ("task out"=w244:refnum<k21>, "error out"=w245:errorcluster)  [unwired: 10 in, 1 out]
    n499 = Select(t=0.0 ("s? t:f"), s=w237, f=w109) -> (s? t:f=w235:dbl)
    n500 = call-poly <vilib>:"DAQmx Write.vi"("task/channels in"=w249, "data"=w235, "error in"=w239) -> ("task out"=w248:refnum<k21>, "error out"=w247:errorcluster)  [unwired: 10 in, 1 out]
    n501 = call <vilib>:"DAQmx Wait Until Done.vi"("task/channels in"=w248, "error in"=w247) -> ("error out"=w246:errorcluster)  [unwired: 12 in, 1 out]
    n502 = call <vilib>:"DAQmx Wait Until Done.vi"("task/channels in"=w244, "error in"=w245) -> ("error out"=w242:errorcluster)  [unwired: 12 in, 1 out]
    n503 = Select(t=w117, s=w63, f=w99) -> (s? t:f=→"calculating error x":dbl)
    n504 = call "swiches.vi"("Numeric 2"=w72, "Numeric"=w71, "Numeric 3"=w73, "Numeric 4"=w74, "Numeric 5"=w75) -> ("xLength"=→"swiches pressed x":dbl, "yLength"=→"swiches pressed y":dbl)  [unwired: 5 in]
  }
  n505 = invoke on="motor 1" class="Slide (strict)" method="Reinit To Default"() -> ()  [unwired: 3 in, 3 out]
  n506 = invoke on="Numeric" class="DigNum (strict)" method="Reinit To Default"() -> ()  [unwired: 3 in, 3 out]
  n507 = invoke on="No of Points" class="DigNum (strict)" method="Reinit To Default"() -> ()  [unwired: 3 in, 3 out]
  n508 = invoke on="Shape drawing steps" class="Enum (strict)" method="Reinit To Default"() -> ()  [unwired: 3 in, 3 out]
  n509 = invoke on="stage circle" class="Enum (strict)" method="Reinit To Default"() -> ()  [unwired: 3 in, 3 out]
  n510 = invoke on="array Y length 2" class="DigNum (strict)" method="Reinit To Default"() -> ()  [unwired: 3 in, 3 out]
  n511 = invoke on="reached x" class="Bool (strict)" method="Reinit To Default"() -> ()  [unwired: 3 in, 3 out]
  n512 = invoke on="array x Length 2" class="DigNum (strict)" method="Reinit To Default"() -> ()  [unwired: 3 in, 3 out]
  n513 = invoke on="Point circle is drawing" class="DigNum (strict)" method="Reinit To Default"() -> ()  [unwired: 3 in, 3 out]
  n514 = invoke on="reached y" class="Bool (strict)" method="Reinit To Default"() -> ()  [unwired: 3 in, 3 out]
  n515 = invoke on="previous index" class="DigNum (strict)" method="Reinit To Default"() -> ()  [unwired: 3 in, 3 out]
  n516 = invoke on="stage rectangle" class="Enum (strict)" method="Reinit To Default"() -> ()  [unwired: 3 in, 3 out]
  n517 = call <vilib>:"Simple Error Handler.vi"("error source (\" \")"="you messed up" ("error source (\" \")"), "error in (no error)"=w48) -> ()  [unwired: 3 in, 5 out]
  n518 = call <vilib>:"Simple Error Handler.vi"("error source (\" \")"="you messed up" ("error source (\" \")"), "error in (no error)"=w45) -> ()  [unwired: 3 in, 5 out]
  n519 = call <vilib>:"DAQmx Clear Task.vi"("task in"=w27, "error in"=w25) -> ()  [unwired: 13 in, 1 out]
  n520 = call <vilib>:"DAQmx Clear Task.vi"("task in"=w17, "error in"=w14) -> ()  [unwired: 13 in, 1 out]
  n521 = call <vilib>:"DAQmx Clear Task.vi"("task in"=w18, "error in"=w15) -> ("error out"=w12:errorcluster)  [unwired: 13 in]
  n522 = call <vilib>:"DAQmx Clear Task.vi"("task in"=w16, "error in"=w13) -> ()  [unwired: 13 in, 1 out]
  n523 = call <vilib>:"Simple Error Handler.vi"("error in (no error)"=w12) -> ()  [unwired: 4 in, 5 out]
  n524 = call <vilib>:"Simple Error Handler.vi"("error source (\" \")"="you messed up" ("error source (\" \")"), "error in (no error)"=w10) -> ()  [unwired: 3 in, 5 out]
